vi "GetWindowPixelDensity.vi"(8 "No Error":errorcluster, 11 "Window [SDL_Window *]":i64) -> (0 "Error Out":errorcluster, 3 "Pixel Density":sgl)   [LabVIEW 2024, in "SDL3.lvlib" / "Video.lvlib"]
doc: "<B>Summary</B>\nGet the pixel density of a window.\n\n<B>Remarks</B>\nThis is a ratio of pixel size to window size. For example, if the window is 1920x1080 and it has a high density back buffer of 3840x2160 pixels, it would have a pixel density of 2.0."
uses:
  Video.lvlib
  Error/Error.lvlib
  Lib/SDL3-32.dll
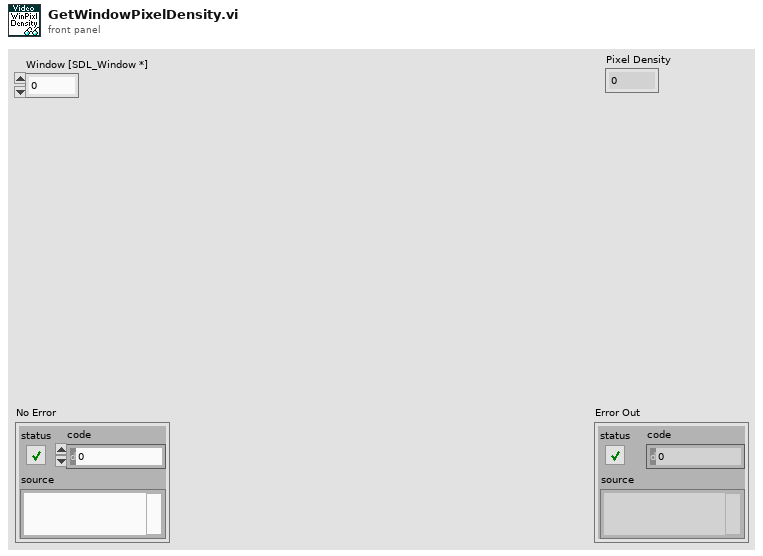
[diagram p1: front panel]
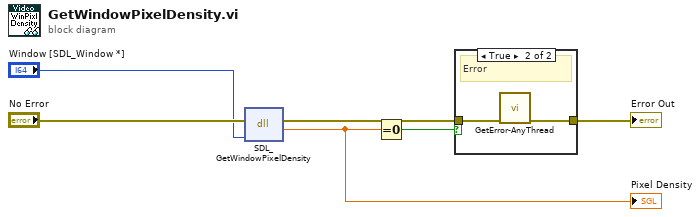
[diagram p0: block diagram]
diagram:
  n1 = dll-call lib="C:/Users/Thomas/Documents/Projects/LV-SDL3/Lib/SDL3-*.*" fn="SDL_GetWindowPixelDensity"(error in="No Error", "window"="Window [SDL_Window *]") -> (error out=w2:errorcluster, "return type"=w3:sgl)  [unwired: 3 in, 1 out]
  "Pixel Density" <- w3
  n2 = Equal To 0?(x=w3) -> (x = 0?=w1:bool)
  n3 = case shown="True" w1 {
    tunnel: w2 -> [w7 w9]
    tunnel: [w7 w8] -> w5
    frame False {
      # "Ok"
    }
    frame True {
      # "Error"
      n4 = call "GetError-AnyThread.vi"("No Error"=w9) -> ("Error Out"=w8:errorcluster)  [unwired: 10 in]
    }
  }
  "Error Out" <- w5
